vi "Generate Ramp.vi"(8 "error in (no error)":errorcluster, 11 "Ramp Use Case In":refnum<class "Ramp Voltage.lvclass">) -> (0 "error out":errorcluster, 3 "Ramp Use Case Out":refnum<class "Ramp Voltage.lvclass">)   [LabVIEW 2020, in "High Level PSU With Tests.lvlib" / "Ramp Voltage.lvclass"]
uses:
  Ramp Voltage.lvclass
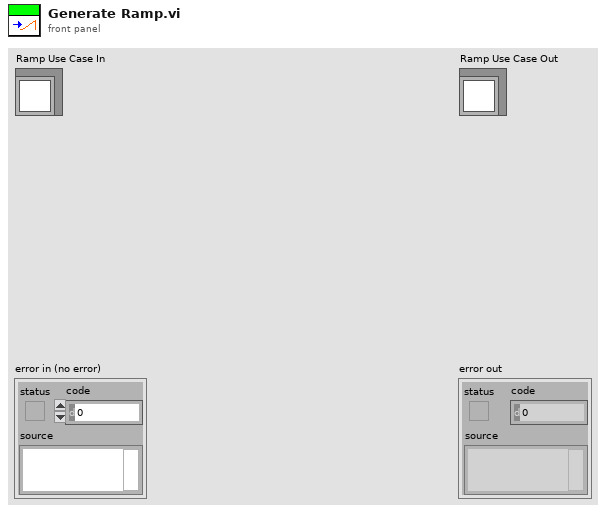
[diagram p1: front panel]
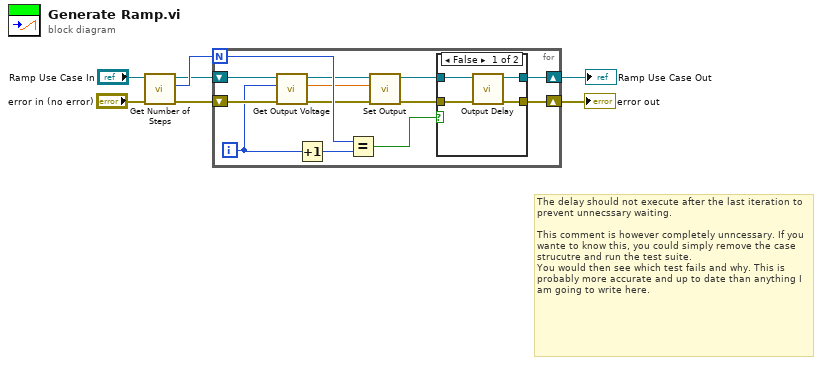
[diagram p0: block diagram]
diagram:
  # "The delay should not execute after the last iteration to prevent unnecssary waiting.\n\nThis comment is however completely unncessary. If you wante to know this, you could simply remove the case strucutre and run the test suite. \nYou would then see which test fails and why. This is probably more accurate and up to date than anything I am going to write here."
  n1 = call "Get Number of Steps.vi"("error in (no error)"="error in (no error)", "Ramp Use Case in"="Ramp Use Case In") -> ("error out"=w1:errorcluster, "Numeric"=w7:i32, "Ramp Use Case out"=w5:refnum<class "Ramp Voltage.lvclass">)  [unwired: 7 in]
  n2 = for {
    N: w7 -> [w16]
    shift-right: [w17] -> w6
    shift-left: w1 -> [w20]
    shift-right: [w19] -> w4
    shift-left: w5 -> [w9]
    i -> [w15]
    n3 = call "Get Output Voltage.vi"("error in (no error)"=w20, "Step index"=w15, "Ramp Use Case in"=w9) -> ("error out"=w12:errorcluster, "Output Voltage [V]"=w11:dbl, "Ramp Use Case in 2"=w10:refnum<class "Ramp Voltage.lvclass">)  [unwired: 6 in]
    n4 = Increment(x=w15) -> (x+1=w14:i32)
    n5 = Equal?(x=w16, y=w14) -> (x = y?=w13:bool)
    n6 = call "Set Output.vi"("error in (no error)"=w12, "Output Voltage [V]"=w11, "Ramp Use Case in"=w10) -> ("error out"=w18:errorcluster, "Ramp Use Case out"=w8:refnum<class "Ramp Voltage.lvclass">)  [unwired: 7 in]
    n7 = case shown="False" w13 {
      tunnel: w8 -> [w24 w25]
      tunnel: [w23 w25] -> w19
      tunnel: w18 -> [w22 w26]
      tunnel: [w21 w26] -> w17
      frame False {
        n8 = call "Output Delay.vi"("error in (no error)"=w22, "Ramp Use Case in"=w24) -> ("error out"=w21:errorcluster, "Ramp Use Case out"=w23:refnum<class "Ramp Voltage.lvclass">)  [unwired: 8 in]
      }
      frame True {
      }
    }
  }
  "error out" <- w6
  "Ramp Use Case Out" <- w4
